vi "Spectrum Merge Pixels v10.5.0.vi"(2 "CCD Area Format":T1, 3 "Raw Spectrum":dbl[](array[numeric])) -> (0 "Spectrum-Array":dbl[][](array[numeric]), 1 "Spectrum-Cluster":T2(array[cluster]))   [LabVIEW 2010]
uses:
  Symphony/TypeDefs/Symphony Area Format.ctl
panel:
  out "Ausgangs-Cluster":T3
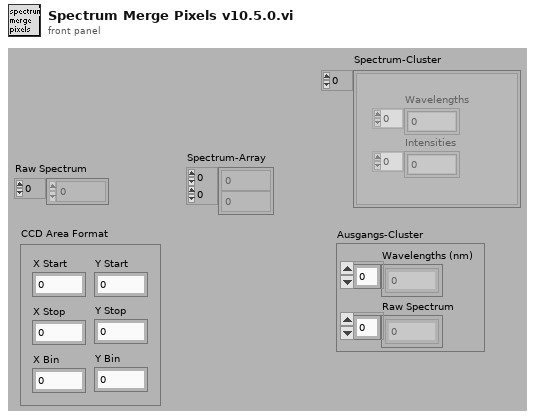
[diagram p1: front panel]
types:
  T1 = typedef "Symphony Area Format.ctl" = cluster{"XStart":i32, "YStart":i32, "XStop":i32, "YStop":i32, "XBin":i32, "YBin":i32}
  T2 = cluster{"Intensities":dbl[], "Wavelengths":dbl[]}[]
  T3 = cluster{"Wavelengths (nm)":dbl[], "Raw Spectrum":dbl[]}
  T4 = cluster{"Axis Out":dbl[], "Raw Spectrum":dbl[]}[]
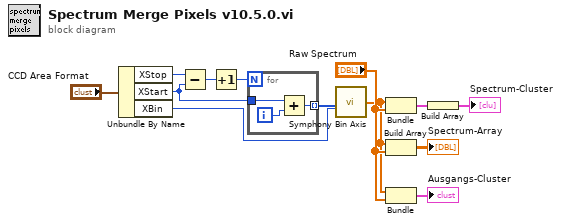
[diagram p0: block diagram]
diagram:
  n1 = Unbundle By Name("CCD Area Format") -> ("XStop"=w6:i32, "XStart"=w5:i32, "XBin"=w2:i32)
  n2 = Subtract(x=w6, y=w5) -> (x-y=w8:i32)
  n3 = Increment(x=w8) -> (x+1=w7:i32)
  n4 = for {
    N: w7 -> [_]
    tunnel: w5 -> [w15]
    tunnel: [w14] -> w3 mode=indexing
    i -> [w16]
    n5 = Add(x=w15, y=w16) -> (x+y=w14:i32)
  }
  n6 = call "Symphony Bin Axis.vi"("Binning Factor"=w2, "Axis In"=w3) -> ("Axis Out"=w1:dbl[])
  n7 = Bundle("Axis Out"=w1, "Raw Spectrum"="Raw Spectrum") -> (w11:cluster{"Axis Out":dbl[], "Raw Spectrum":dbl[]})  [unwired: 1 in]
  n8 = Build Array(w1, "Raw Spectrum") -> (→"Spectrum-Array":dbl[][])
  n9 = Bundle("Axis Out"=w1, "Raw Spectrum"="Raw Spectrum") -> (→"Ausgangs-Cluster":cluster{"Axis Out":dbl[], "Raw Spectrum":dbl[]})  [unwired: 1 in]
  n10 = Build Array(w11) -> (→"Spectrum-Cluster":T4)
